vi "Get Named Range.vi"(7 "Sheet Name":string, 8 "error in":errorcluster, 10 "Range Identifier":string, 11 "SpreadsheetDoc in":refnum<k24>) -> (0 "error out":errorcluster, 2 "Range":string, 3 "SpreadsheetDoc out":refnum<k24>, 5 "Sheet Name":string)   [LabVIEW 2019, in "Open Xml.lvlib"]
uses:
  Open Xml.lvlib
  D:/git/Open-Xml-LabVIEW/Source/DocumentFormat.OpenXml.dll
  DocumentFormat.OpenXml.dll
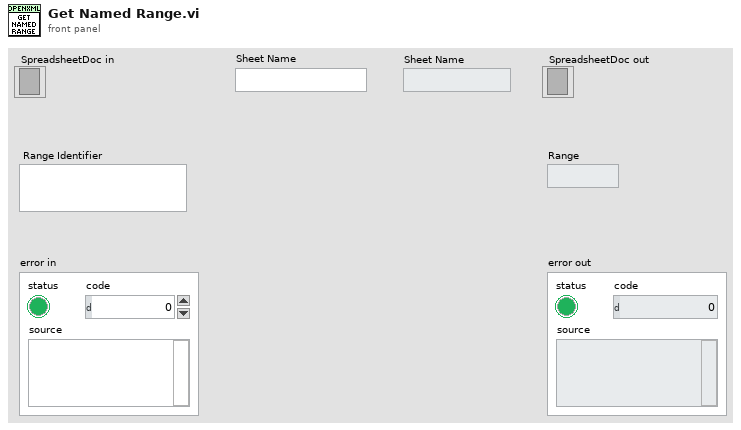
[diagram p1: front panel]
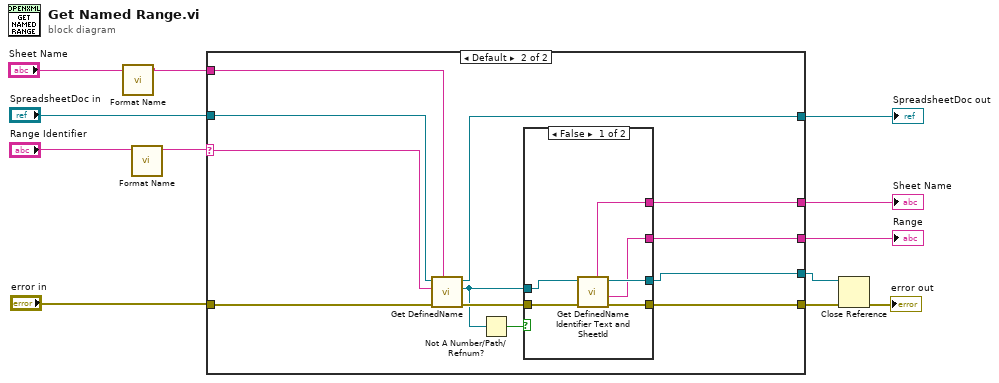
[diagram p0: block diagram]
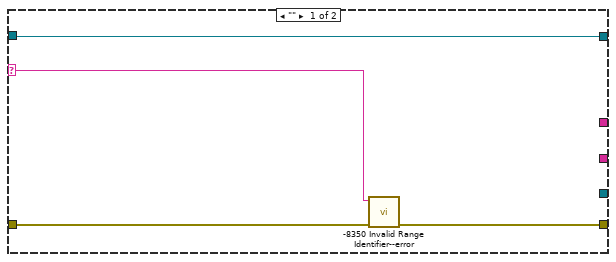
[diagram p2: hidden frame]
diagram:
  n1 = call "Format Name.vi"("Sheet Name"="Sheet Name") -> ("Formatted Sheet Name"=w1:string)  [unwired: 10 in]
  n2 = call "Format Name.vi"("Sheet Name"="Range Identifier") -> ("Formatted Sheet Name"=w4:string)  [unwired: 10 in]
  n3 = case shown="Default" w4 {
    selector: w4 -> [w14 w26]
    tunnel: "error in" -> [w16 w28]
    tunnel: [w15 w19] -> w12
    tunnel: "SpreadsheetDoc in" -> [w13 w22]
    tunnel: [w13 w21] -> w10
    tunnel: w1 -> [_ w27]
    tunnel: [_ w20] -> w9
    tunnel: [_ w18] -> w8
    tunnel: [_ w17] -> w7
    frame "" {
      n4 = call "-8350 Invalid Range Identifier--error.vi"("error in"=w16, "Argument"=w14) -> ("error out"=w15:errorcluster)  [unwired: 9 in]
    }
    frame Default {
      n5 = call "Get DefinedName.vi"("Sheet Name"=w27, "error in"=w28, "Range Identifier"=w26, "SpreadsheetDoc in"=w22) -> ("error out"=w25:errorcluster, "DefinedName"=w23:refnum<k24>, "SpreadsheetDoc out"=w21:refnum<k24>)  [unwired: 4 in, 1 out]
      n6 = Not A Number/Path/Refnum?(number/path/refnum=w23) -> (NaN/Path/Refnum?=w24:bool)
      n7 = case shown="False" w24 {
        tunnel: [w34 w35] -> w17
        tunnel: w25 -> [w32 w36]
        tunnel: w23 -> [w33 w35]
        tunnel: [w31 w36] -> w19
        tunnel: [w30 _] -> w20
        tunnel: [w29 _] -> w18
        frame False {
          n8 = call "Get DefinedName Identifier Text and SheetId.vi"("error in"=w32, "DefinedName in"=w33) -> ("error out"=w31:errorcluster, "Range"=w29:string, "DefinedName out"=w34:refnum<k24>, "Sheet Name"=w30:string)  [unwired: 5 in, 1 out]
        }
        frame True {
        }
      }
    }
  }
  "SpreadsheetDoc out" <- w10
  "Sheet Name" <- w9
  "Range" <- w8
  n9 = Close Reference(reference=w7, error in (no error)=w12) -> (error out=→"error out":errorcluster)
